vi "CPU_FM_Demodulate_CDB.vi"(8 "error in (no error)":errorcluster, 11 "1D_CDB in":cdb[](array[numeric])) -> (0 "error out":errorcluster, 3 "1D_DBL out":dbl[](array[numeric]), 4 "dt":dbl format="%#_6p")   [LabVIEW 2020]
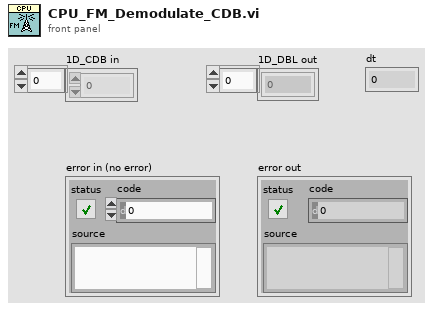
[diagram p1: front panel]
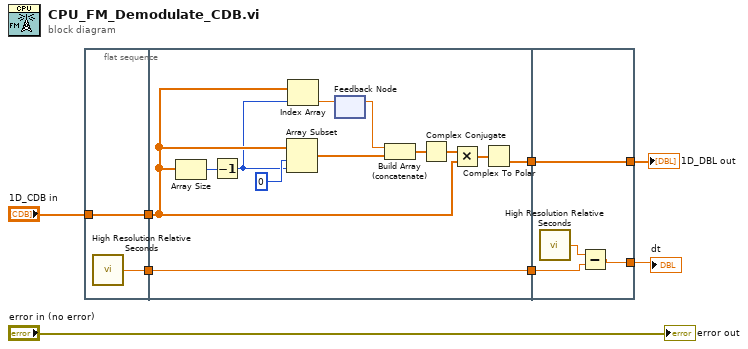
[diagram p0: block diagram]
diagram:
  n1 = flat-sequence {
    tunnel: "1D_CDB in" -> [w10]
    tunnel: [w10] -> w5
    tunnel: [w9] -> w3
    tunnel: w5 -> [w16]
    tunnel: [w22] -> w4
    tunnel: w3 -> [w17]
    tunnel: [w17] -> w2
    tunnel: [w26] -> w7
    tunnel: w4 -> [w26]
    tunnel: w2 -> [w24]
    tunnel: [w23] -> w1
    frame #0 {
      n2 = call <vilib>:"High Resolution Relative Seconds.vi"() -> ("relative seconds"=w9:dbl)
    }
    frame #1 {
      n3 = Array Size(array=w16) -> (size(s)=w20:i32)
      n4 = Decrement(x=w20) -> (x-1=w15:i32)
      n5 = Array Subset(array=w16, index=0, length=w15) -> (w13:cdb[])
      n6 = Index Array(array=w16, index=w15) -> (element=w14:cdb)
      n7 = feedback #1() -> (w12:cdb)  [unwired: 1 in]
      n8 = feedback-in #1(w14) -> ()
      n9 = Build Array (concatenate)(w12, w13) -> (w11:cdb[])
      n10 = Complex Conjugate(1:w11) -> (0:w19:cdb[])
      n11 = Multiply(x=w19, y=w16) -> (x*y=w21:cdb[])
      n12 = Complex To Polar(r * e^(i*theta)=w21) -> (theta=w22:dbl[])  [unwired: 1 out]
    }
    frame #2 {
      n13 = call <vilib>:"High Resolution Relative Seconds.vi"() -> ("relative seconds"=w25:dbl)
      n14 = Subtract(x=w25, y=w24) -> (x-y=w23:dbl)
    }
  }
  "1D_DBL out" <- w7
  "error out" <- "error in (no error)"
  "dt" <- w1
